vi "Create StandardText Paragraph.vi"(8 "error in (no error)":errorcluster, 11 "ooWriter in":refnum<class "ooWriter.lvclass">) -> (0 "error out":errorcluster, 2 "StandardTextParagraph":refnum<k24>, 3 "ooWriter out":refnum<class "ooWriter.lvclass">)   [LabVIEW 2009, in "ooWriter.lvclass"]
uses:
  ooWriter.lvclass
  C:/Projets/LAVAG/OpenOfficeRGT/AODL/DLLs/AODL.dll
  ooWriter.lvclass/ooWriter.ctl
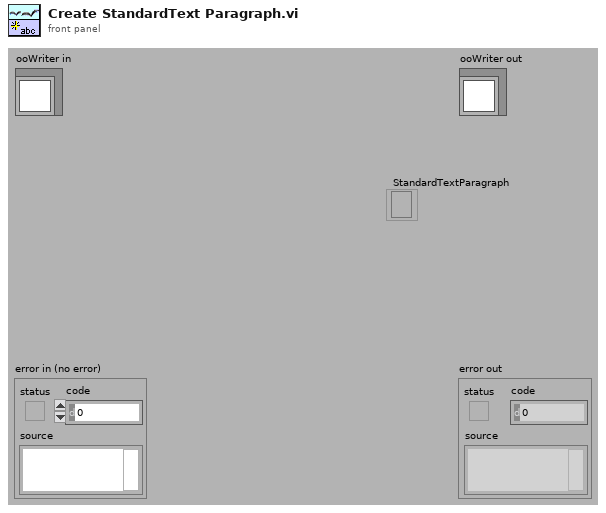
[diagram p1: front panel]
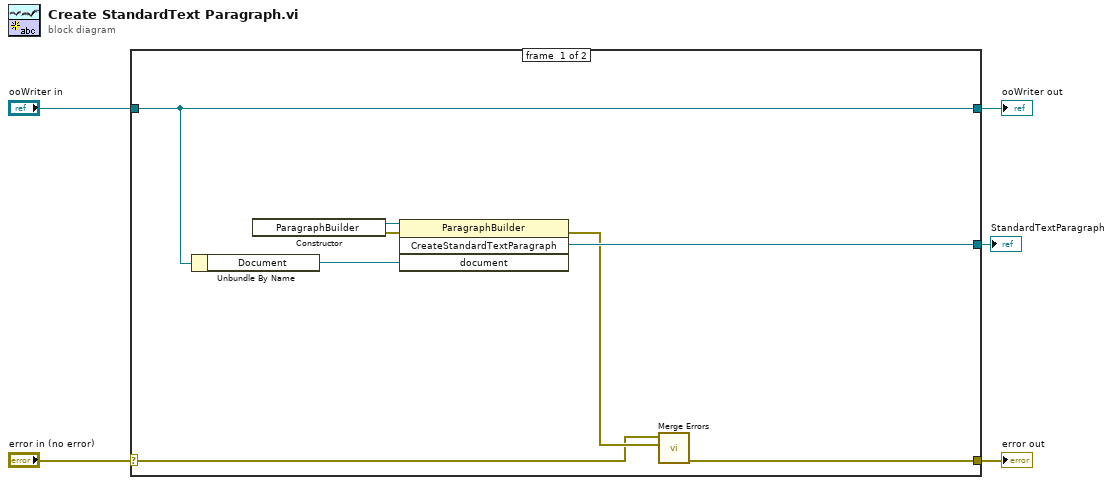
[diagram p0: block diagram]
diagram:
  n1 = case shown="No Error" "error in (no error)" {
    selector: "error in (no error)" -> [w7 w15]
    tunnel: [w6 w15] -> w4
    tunnel: [w11 w14] -> w2
    tunnel: "ooWriter in" -> [w11 w14]
    tunnel: [w9 _] -> w1
    frame #0 {
      n2 = Unbundle By Name(w11) -> ("Document"=w10:refnum<k24>)
      n3 = constructor class="ParagraphBuilder"() -> (reference out=w12:refnum<k24>, error out=w13:errorcluster)  [unwired: 3 in, 1 out]
      n4 = invoke class="ParagraphBuilder" method="CreateStandardTextParagraph"(reference=w12, error in=w13, "document"=w10) -> (error out=w8:errorcluster, "CreateStandardTextParagraph"=w9:refnum<k24>)  [unwired: 1 in, 2 out]
      n5 = call <vilib>:"Merge Errors.vi"("error in 2 (no error)"=w8, "error in 1 (no error)"=w7) -> ("error out"=w6:errorcluster)  [unwired: 5 in]
    }
    frame #1 {
    }
  }
  "error out" <- w4
  "ooWriter out" <- w2
  "StandardTextParagraph" <- w1
